vi "Working with defaults for Variants.vi"() -> ()   [LabVIEW 2015]
uses:
  <vilib>/NI/JSON Support for LabVIEW/JSON Data Classes/JSON Object/Insert Key Value Pair.vi
  <vilib>/NI/JSON Support for LabVIEW/JSON Data Classes/JSON Object/Insert Key Value Pair (Single Numeric).vi
  <vilib>/NI/JSON Support for LabVIEW/JSON Data Classes/JSON Object/Insert Key Value Pair (Single String).vi
  <vilib>/NI/JSON Support for LabVIEW/JSON Data Classes/JSON Object/JSON Object.lvclass
  <vilib>/NI/JSON Support for LabVIEW/JSON Data Classes/JSON Object/Set Object Parameters XNode/Set Object Parameters.xnode
  <vilib>/NI/JSON Support for LabVIEW/JSON Data Classes/JSON Helper/JSON Helper.lvclass
panel:
  out "data":T1
  out "defaulted keys":string[](array[string])
  in  "Defaults":T1
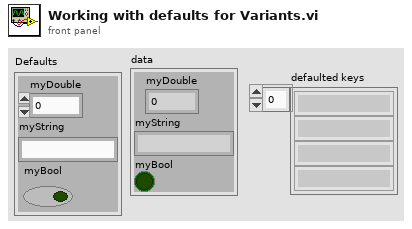
[diagram p1: front panel]
types:
  T1 = cluster{"myDouble":dbl, "myString":string, "myBool":bool}
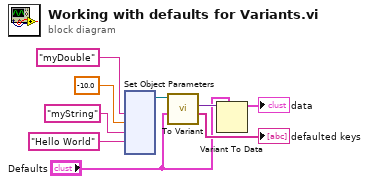
[diagram p0: block diagram]
diagram:
  n1 = xnode "Set Object Parameters"("key"="myDouble", "key"="myString", "parameter"=-10.0, "parameter"="Hello World") -> ("JSON Object Out"=w5:refnum<class "JSON Object.lvclass">)  [unwired: 2 in, 3 out]
  n2 = call <vilib>:"To Variant.vi"("datatype and defaults"="Defaults", "JSON Datatype in"=w5) -> ("defaulted keys"=→"defaulted keys":string[], "Variant"=w3:variant)  [unwired: 7 in, 1 out]
  n3 = Variant To Data(type="Defaults", Variant=w3) -> (data=→"data":T1)  [unwired: 1 in, 1 out]
